vi "UDP Data Link - Configuration Utilities - Get Tx Channels Groups Information.vi"(8 "error in":errorcluster, 11 "Selected Channel Refs":T2[](array[typedef]) format="%.0x") -> (0 "error out":errorcluster, 3 "Channels":T1[](array[typedef]) {"Data Type" items=["U8", "U16", "U32", "U64", "I8", "I16", "I32", "I64", "SGL", "DBL", "EXT"]})   [LabVIEW 2012, in "UDP Data Link System Explorer.lvlib"]
doc: "Gets channel path, unit, and description."
uses:
  UDP Data Link System Explorer.lvlib
  <vilib>/NI Veristand/Custom Device API/Custom Device Item Ref.ctl
  TypeDefs/UDP Data Link - TypeDefs - XML Channel.ctl
  <vilib>/NI Veristand/Custom Device API/Custom Device API.lvlib
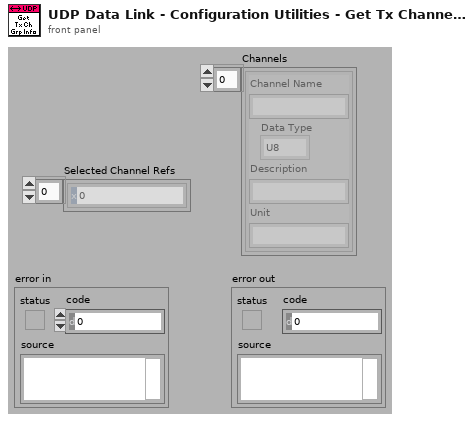
[diagram p1: front panel]
types:
  T1 = typedef "UDP Data Link System Explorer.lvlib/UDP Data Link - TypeDefs - XML Channel.ctl" = cluster{"Channel Name":string, "Data Type":u16, "Description":string, "Unit":string}
  T2 = typedef "Custom Device API.lvlib/Custom Device Item Ref.ctl" = u64
  T3 = typedef "Custom Device API.lvlib/Custom Device Channel.ctl" = cluster{"Type":T4, "Units":string, "Default Value":dbl, "Faultable":bool, "Scalable":bool}
  T4 = typedef "Custom Device API.lvlib/Custom Device Channel Type.ctl" = enum16{"Input", "Output"}
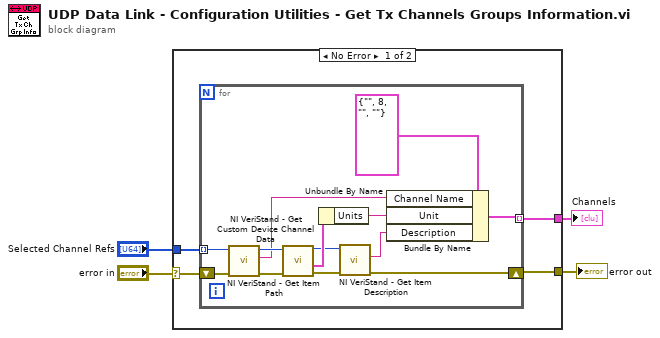
[diagram p0: block diagram]
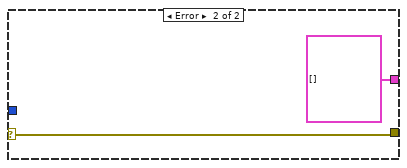
[diagram p2: hidden frame]
diagram:
  n1 = case shown="No Error" "error in" {
    selector: "error in" -> [w6 w23]
    tunnel: "Selected Channel Refs" -> [w8 _]
    tunnel: [w7 w23] -> w3
    tunnel: [w5 T1[] []] -> w1
    frame No Error {
      n2 = for {
        shift-right: [w17] -> w7
        shift-left: w6 -> [w13]
        tunnel: w8 -> [w12] mode=indexing
        tunnel: [w15] -> w5 mode=indexing
        n3 = call <vilib>:"NI VeriStand - Get Item Path.vi"("error in (no error)"=w13, "Item Ref in"=w12) -> ("error out"=w14:errorcluster, "Path"=w10:string, "Item Ref out"=w11:T2)  [unwired: 6 in, 1 out]
        n4 = call <vilib>:"NI VeriStand - Get Custom Device Channel Data.vi"("error in (no error)"=w14, "Channel Ref in"=w11) -> ("error out"=w18:errorcluster, "Channel"=w21:T3, "Channel Ref out"=w19:T2)  [unwired: 4 in, 3 out]
        n5 = Unbundle By Name(w21) -> ("Units"=w20:string)
        n6 = call <vilib>:"NI VeriStand - Get Item Description.vi"("error in (no error)"=w18, "Item Ref in"=w19) -> ("error out"=w17:errorcluster, "Description"=w16:string)  [unwired: 6 in, 2 out]
        n7 = Bundle By Name(cluster=T1 {"Channel Name"="", "Data Type"=8, "Description"="", "Unit"=""} ("Channel"), "Channel Name"=w10, "Unit"=w20, "Description"=w16) -> (w15:T1)
      }
    }
    frame Error {
    }
  }
  "error out" <- w3
  "Channels" <- w1
